vi "HandsOnGlobals.vi"() -> ()   [LabVIEW 2020]
panel:
  out "PWMFreq":dbl
  out "PWMDuty":dbl
  out "DI 4 Pressed":bool
  out "DI 3 Pressed":bool
  out "DI 2 Pressed":bool
  out "DI 1 Pressed":bool
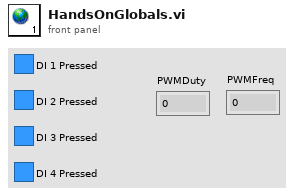
[diagram p1: front panel]
diagram:
